vi "DFT_noisewaveform.vi"() -> (0 "Noise density":dbl[](graph))   [LabVIEW 2013]
uses:
  <vilib>/Analysis/4window.llb/windowTd.ctl
  <vilib>/measure/maspectr.llb/Power Spectrum and PSD Export Mode.ctl
  <vilib>/measure/maresamp.llb/Resample Waveform (single shot).vi
  <vilib>/Analysis/baseanly.llb/Inverse f Filter (DBL).vi
  <vilib>/measure/maspectr.llb/FFT Power Spectrum and PSD for 1 Chan.vi
  <vilib>/Analysis/NI_AALPro.lvlib
  <vilib>/measure/NI_MAPro.lvlib
  <vilib>/measure/NI_MABase.lvlib
  <vilib>/Analysis/NI_AALBase.lvlib
panel:
  in  "exponent":dbl=1.0 format="%.2p"
  in  "dB On (F)":bool=TRUE
  in  "filter specifications":T1={"lower cutoff freq"=0.01, "higher cutoff freq"=400.0, "order"=5}
  out "Waveform":waveform(dbl)(graph)
  in  "sampling info":cluster{"Fs":dbl, "#s":dbl}={"Fs"=1000.0, "#s"=10000.0} {"#s" format="%#.6g"; "Fs" format="%#.6g"}
  out "Power Spectral Density":cluster{"f0":dbl, "df":dbl, "magnitude":dbl[]}(graph)
  in  "noise type":T2(ring)=enum."inverse f"
  in  "noise amplitude":dbl=0.1 format="%#.6g"
  in  "Stop":bool
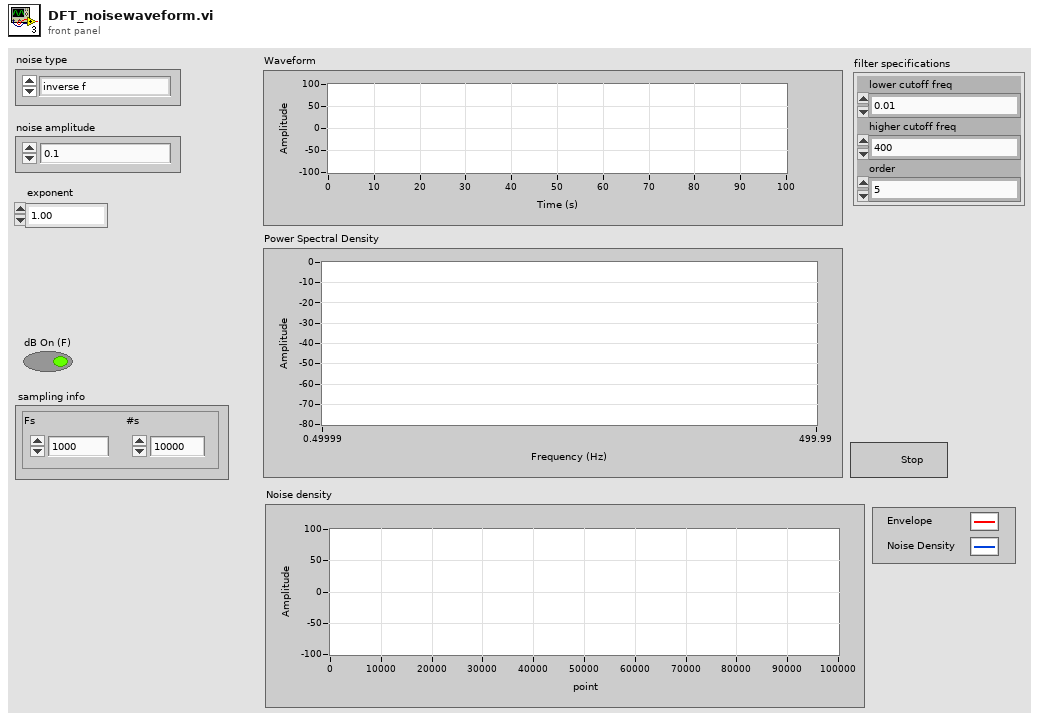
[diagram p1: front panel]
types:
  T1 = cluster{"lower cutoff freq":dbl, "higher cutoff freq":dbl, "order":i32}
  T2 = enum16{"uniform white", "Gaussian white", "periodic", "inverse f"}
  T3 = cluster{"averaging mode":enum16{"No averaging", "Vector averaging", "RMS averaging", "Peak hold"}, "weighting mode":enum16{"Linear", "Exponential"}, "number of averages":u32}
  T4 = typedef "NI_MAPro.lvlib/Power Spectrum and PSD Export Mode.ctl" = u16
  T5 = typedef "NI_AALPro.lvlib/windowTd.ctl" = u32
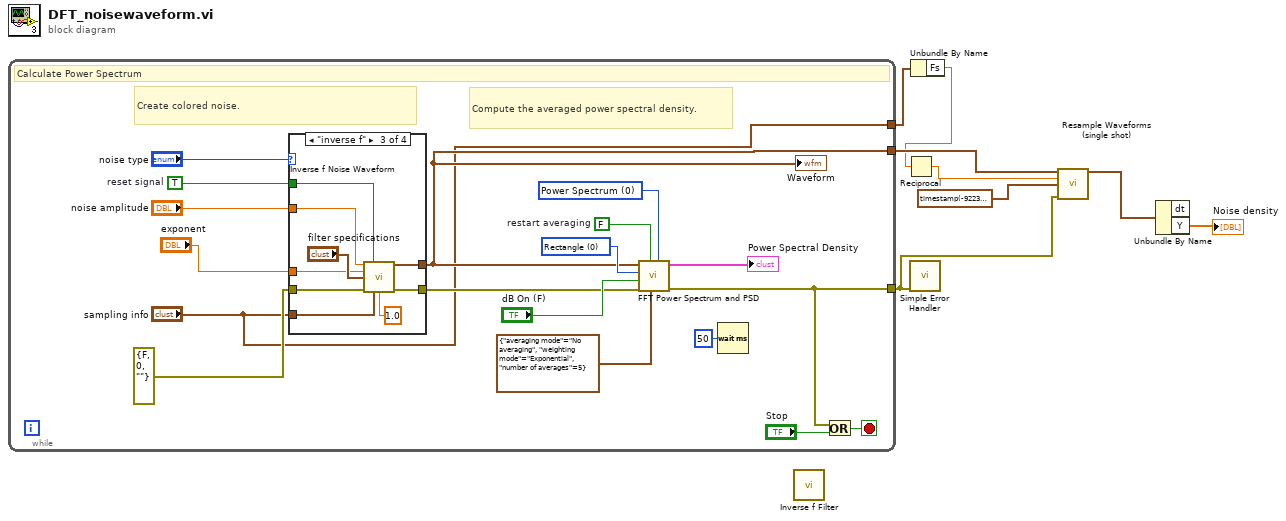
[diagram p0: block diagram]
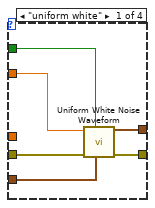
[diagram p2: hidden frame]
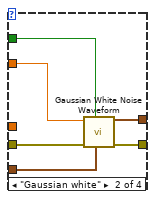
[diagram p3: hidden frame]
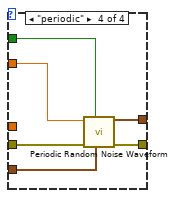
[diagram p4: hidden frame]
diagram:
  n1 = while {
    tunnel: [w14] -> w3
    tunnel: [w10] -> w8
    tunnel: ["sampling info"] -> w7
    stop <- w15 stop-if-true
    w16 = T4 0 items=["Power Spectrum", "Power Spectral Density"] ("export mode")
    w17 = T5 0 items=["Rectangle"=0, "Hanning"=1, "Hamming"=2, "Blackman-Harris"=3, "Exact Blackman"=4, "Blackman"=5, "Flat Top"=6, "4 Term B-Harris "=7, "7 Term B-Harris"=8, "Low Sidelobe"=9, "Blackman Nuttall"=11, "Triangle"=30, "Bartlett-Hanning"=31, "Bohman"=32, "Parzen"=33, "Welch"=34, "Kaiser"=60, "Dolph-Chebyshev"=61, "Gaussian"=62] ("window")
    w24 = TRUE  # reset signal
    w25 = FALSE  # restart averaging
    # "Compute the averaged power spectral density."
    # "Create colored noise."
    # "Calculate Power Spectrum"
    n2 = case shown="\"inverse f\"" "noise type" {
      tunnel: errorcluster {"status"=FALSE, "code"=0, "source"=""} ("error out") -> [w32 w38 w47 w53]
      tunnel: "sampling info" -> [w31 w37 w46 w52]
      tunnel: w24 -> [w30 w36 w45 w48]
      tunnel: "noise amplitude" -> [w29 w35 w44 w51]
      tunnel: [w28 w34 w43 w50] -> w10
      tunnel: [w27 w33 w42 w49] -> w12
      tunnel: "exponent" -> [_ _ w40 _]
      frame "uniform white" {
        n3 = call <vilib>:"Uniform White Noise Waveform.vi"("sampling info"=w31, "reset signal"=w30, "error in (no error)"=w32, "amplitude"=w29) -> ("error out"=w27:errorcluster, "signal out"=w28:waveform(dbl))  [unwired: 6 in]
      }
      frame "Gaussian white" {
        n4 = call <vilib>:"Gaussian White Noise Waveform.vi"("sampling info"=w37, "reset signal"=w36, "error in (no error)"=w38, "standard deviation"=w35) -> ("error out"=w33:errorcluster, "signal out"=w34:waveform(dbl))  [unwired: 6 in]
      }
      frame "inverse f" {
        n5 = call <vilib>:"Inverse f Noise Waveform.vi"("noise density"=w44, "reset signal (F)"=w45, "exponent"=w40, "filter specifications"="filter specifications", "error in (no error)"=w47, "sampling info"=w46, "reference freq (Hz)"=1.0) -> ("signal out"=w43:waveform(dbl), "error out"=w42:errorcluster)  [unwired: 4 in, 3 out]
      }
      frame "periodic" {
        n6 = call <vilib>:"Periodic Random Noise Waveform.vi"("sampling info"=w52, "reset signal"=w48, "error in (no error)"=w53, "spectral amplitude"=w51) -> ("error out"=w49:errorcluster, "signal out"=w50:waveform(dbl))  [unwired: 6 in]
      }
    }
    "Waveform" <- w10
    n7 = call-poly <vilib>:"FFT Power Spectrum and PSD.vi"("export mode"=w16, "averaging parameters"=T3 {"averaging mode"=enum."No averaging", "weighting mode"=enum."Exponential", "number of averages"=5}, "restart averaging (F)"=w25, "error in (no error)"=w12, "dB On (F)"="dB On (F)", "window"=w17, "time signal"=w10) -> ("error out"=w14:errorcluster, "Power Spectrum / PSD"=→"Power Spectral Density":cluster{"f0":dbl, "df":dbl, "magnitude":dbl[]})  [unwired: 1 in, 2 out]
    n8 = Wait (ms)(milliseconds to wait=u32 50) -> ()  [unwired: 1 out]
    n9 = Or(x=w14, y="Stop") -> (x .or. y?=w15:bool)
  }
  n10 = call-poly <vilib>:"Inverse f Filter.vi"() -> ()  [unwired: 7 in, 5 out]
  n11 = call <vilib>:"Simple Error Handler.vi"("error in (no error)"=w3) -> ()  [unwired: 4 in, 5 out]
  n12 = Unbundle By Name(w7) -> ("Fs"=w5:dbl)
  n13 = Reciprocal(x=w5) -> (1/x=w6:dbl)
  n14 = call-poly <vilib>:"Resample Waveforms (single shot).vi"("waveform in"=w8, "dt"=w6, "t0"=timestamp(-9223372036854775808 s since 1904-01-01), "error in (no error)"=w3) -> ("resampled waveform out"=w2:waveform(dbl))  [unwired: 8 in, 3 out]
  n15 = Unbundle By Name(w2) -> ("Y"=→"Noise density":dbl[])  [unwired: 1 out]
